vi "Control Panel.vi"(8 "error in (no error)":errorcluster, 11 "Fake Analog Output in":refnum<class "Analog Output.lvclass">) -> (0 "error out":errorcluster, 3 "Fake Analog Output out":refnum<class "Analog Output.lvclass">)   [LabVIEW 2017, in "Analog Output.lvclass"]
doc: "(Dynamic) A user-level application that simulates the physical front panel of the Instrument. Provide the user with buttons to manually control features of the instrument, and provide indicators of its current state."
uses:
  Analog Output.lvclass
  Analog Output.lvclass/Analog Output.ctl
  <vilib>/DAQmx/write.llb/DAQmx Write (Analog DBL 1Chan 1Samp).vi
  <vilib>/DAQmx/miscellaneous.llb/DAQmx Fill In Error Info.vi
  Utility Classes/Scannable/Scannable.lvclass
  <resource>/objmgr/daqmx.rc
panel:
  in  "Copy actual to set":bool
  in  "Populate fields with member data":bool
  out "Ch1 voltage":dbl[unit]
  out "Ch1 lower limit":dbl[unit]
  out "Ch1 upper limit":dbl[unit]
  out "Ch0 voltage":dbl[unit]
  out "Ch0 lower limit":dbl[unit]
  out "Ch0 upper limit":dbl[unit]
  in  "Set Ch1 Voltage":bool
  in  "Set Ch0 Voltage":bool
  in  "Ch1 voltage set":dbl[unit]
  in  "Ch1 lower limit set":dbl[unit]
  in  "Ch1 upper limit set":dbl[unit]
  in  "Ch0 voltage set":dbl[unit]
  in  "Ch0 lower limit set":dbl[unit]
  in  "Ch0 upper limit set":dbl[unit]
  in  "Set Parameters":bool
  in  "Read to Control":bool
  in  "Read Parameters":bool
  in  "stop":bool
  # "We cannot read in the currently set voltage values !"
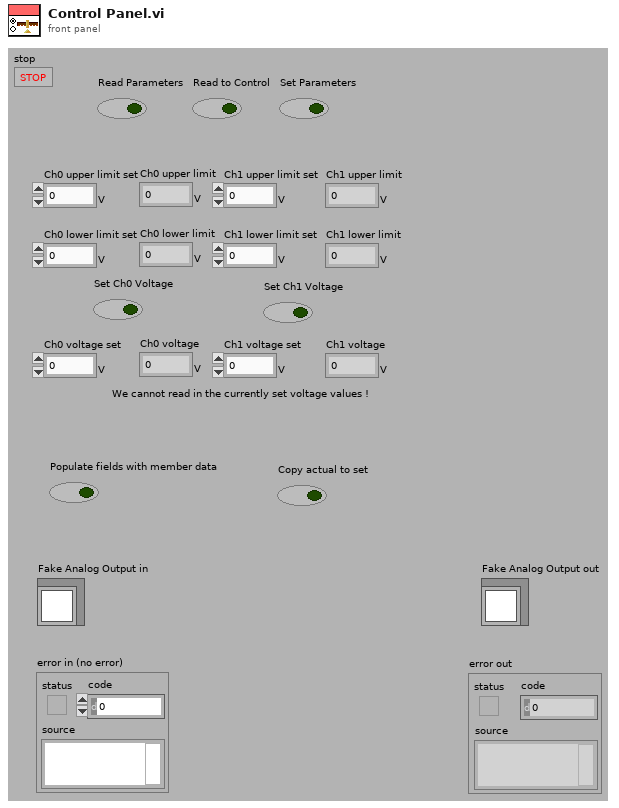
[diagram p1: front panel]
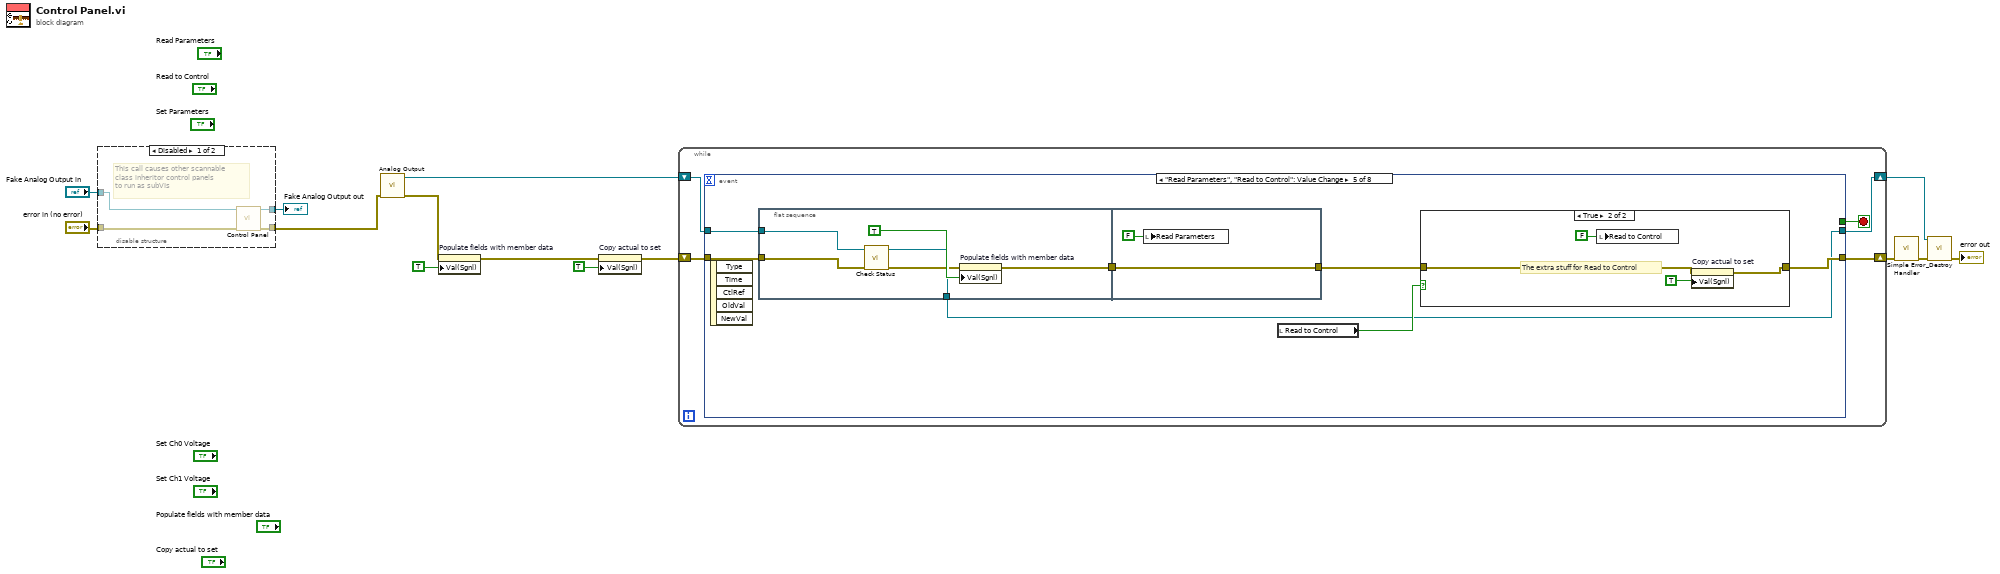
[diagram p0: block diagram]
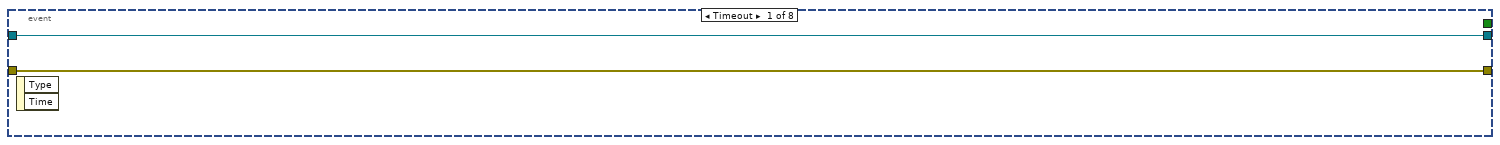
[diagram p3: hidden frame]
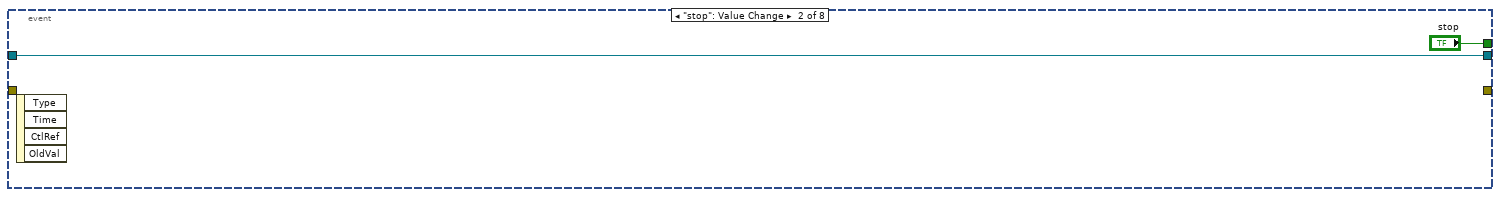
[diagram p4: hidden frame]
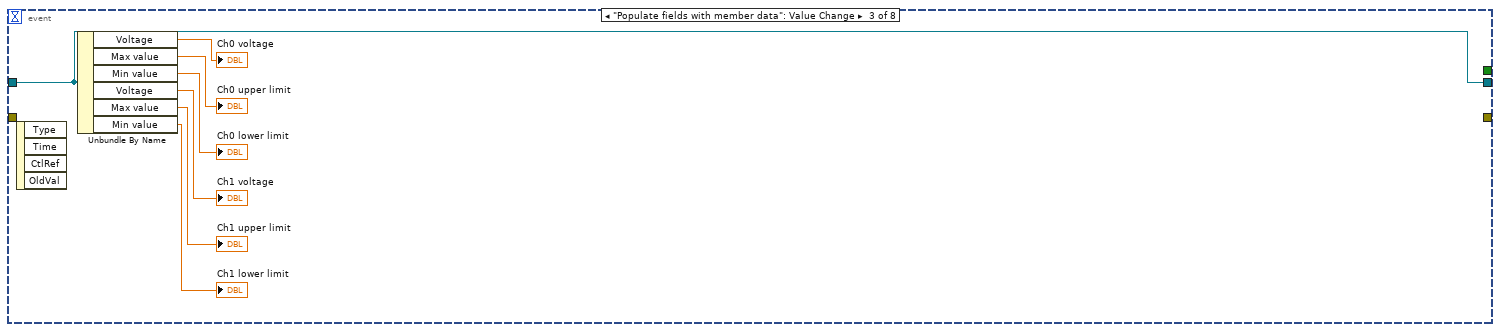
[diagram p5: hidden frame]
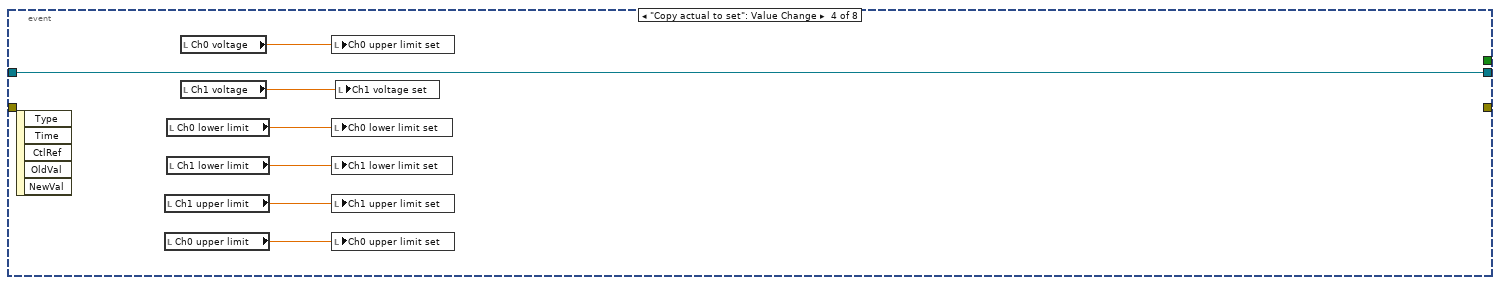
[diagram p6: hidden frame]
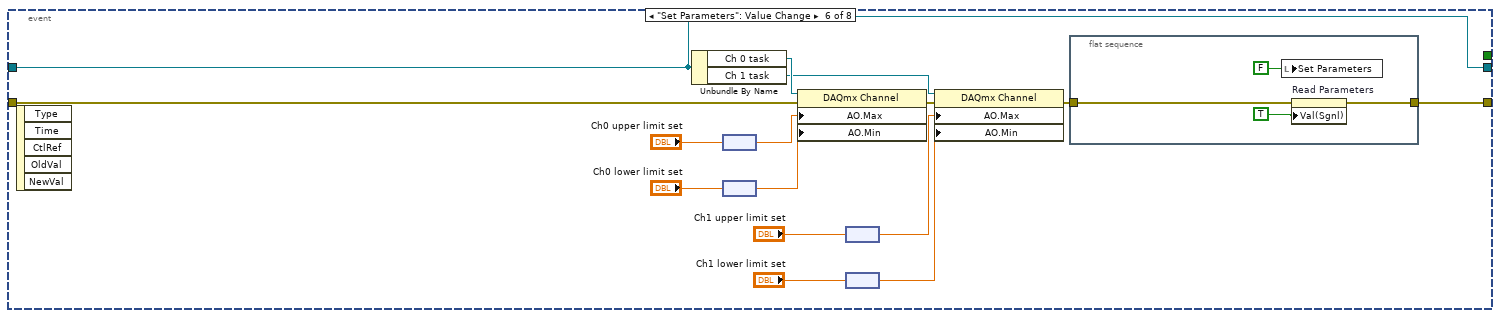
[diagram p8: hidden frame]
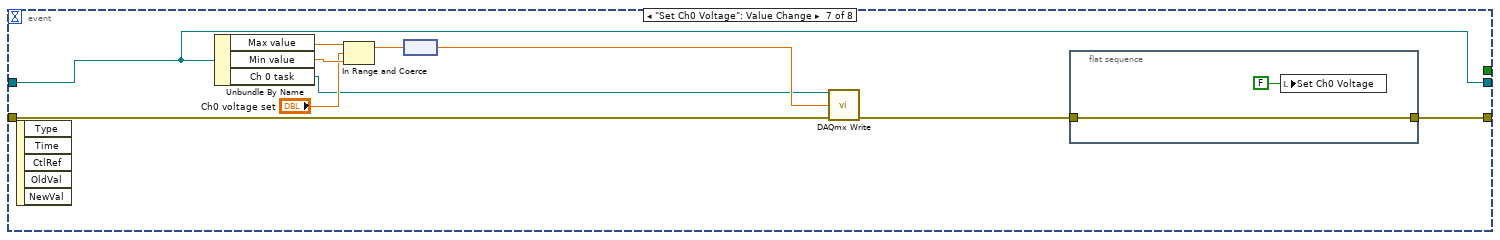
[diagram p9: hidden frame]
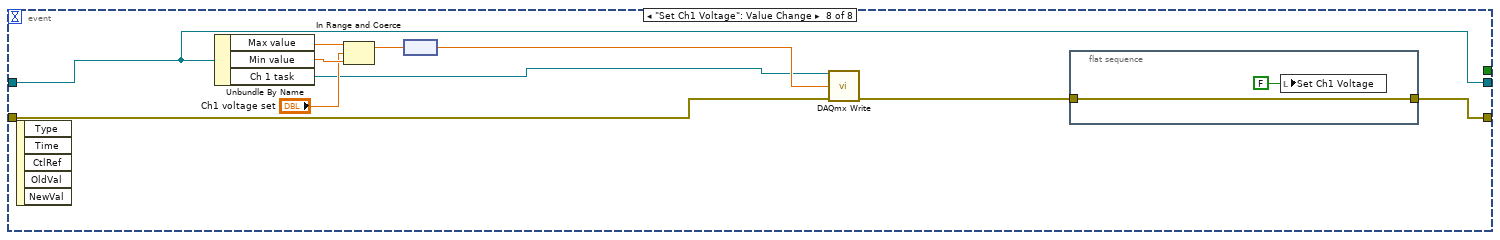
[diagram p10: hidden frame]
diagram:
  n1 = disable-structure shown="Disabled" {
    disable-tunnel: [w18 w20] -> w14
    disable-tunnel: "error in (no error)" -> [w17 w19]
    disable-tunnel: "Fake Analog Output in" -> [w16 w20]
    disable-tunnel: [w15 w19] -> w11
    frame Disabled {
      # "This call causes other scannable\nclass inheritor control panels\nto run as subVIs"
      n2 = call-parent "Control Panel.vi"("error in (no error)"=w17, "Instrument in"=w16) -> ("error out"=w15:errorcluster, "Instrument out"=w18:refnum<class "Analog Output.lvclass">)  [unwired: 8 in]
    }
    frame Enabled {
    }
  }
  "Fake Analog Output out" <- w14
  n3 = call "Analog Output.vi"("error in (no error)"=w11) -> ("error out"=w9:errorcluster, "Analog Output out"=w3:refnum<class "Analog Output.lvclass">)  [unwired: 9 in]
  n4 = property on="Populate fields with member data" class="Bool (strict)"(error in=w9, "Val(Sgnl)"=TRUE ("Value (Signaling)")) -> (error out=w7:errorcluster)  [unwired: 1 in, 1 out]
  n5 = property on="Copy actual to set" class="Bool (strict)"(error in=w7, "Val(Sgnl)"=TRUE ("Value (Signaling)")) -> (error out=w6:errorcluster)  [unwired: 1 in, 1 out]
  n6 = while {
    shift-right: [w23] -> w2
    shift-left: w3 -> [w24]
    shift-right: [w22] -> w1
    shift-left: w6 -> [w25]
    stop <- w21 stop-if-true
    n7 = event shown="[4] \"Read Parameters\", \"Read to Control\": Value Change" {
      selector: _ -> [_ _ _ _ _ _ _ _]
      dyn-events: _ -> [_ _ _ _ _ _ _ _]
      timeout: _ -> [_ _ _ _ _ _ _ _]
      tunnel: [w27 _ _ _ w45 w69 w91 w103] -> w22
      tunnel: w25 -> [w27 _ _ _ w49 w78 w85 w97]
      tunnel: w24 -> [w26 w28 w36 w37 w50 w68 w90 w98]
      tunnel: [w26 w28 w36 w37 w44 w68 w90 w98] -> w23
      tunnel: [_ "stop" _ _ _ _ _ _] -> w21
      event Timeout {
        n8 = event-data() -> ()  [unwired: 1 in, 2 out]
      }
      event "stop": Value Change {
        n9 = event-data() -> ()  [unwired: 1 in, 4 out]
      }
      event "Populate fields with member data": Value Change {
        n10 = event-data() -> ()  [unwired: 1 in, 4 out]
        n11 = Unbundle By Name(w36) -> ("Voltage"=→"Ch0 voltage":dbl[unit], "Max value"=→"Ch0 upper limit":dbl[unit], "Min value"=→"Ch0 lower limit":dbl[unit], "Voltage"=→"Ch1 voltage":dbl[unit], "Max value"=→"Ch1 upper limit":dbl[unit], "Min value"=→"Ch1 lower limit":dbl[unit])
      }
      event "Copy actual to set": Value Change {
        n12 = event-data() -> ()  [unwired: 1 in, 5 out]
        n13 = local read "Ch1 upper limit"() -> (w39:dbl[unit])
        n14 = local read "Ch0 upper limit"() -> (w42:dbl[unit])
        n15 = local read "Ch0 lower limit"() -> (w43:dbl[unit])
        n16 = local read "Ch1 lower limit"() -> (w40:dbl[unit])
        n17 = local read "Ch0 voltage"() -> (w41:dbl[unit])
        n18 = local read "Ch1 voltage"() -> (w38:dbl[unit])
        n19 = local write "Ch0 upper limit set"(w41) -> ()
        n20 = local write "Ch0 lower limit set"(w43) -> ()
        n21 = local write "Ch1 lower limit set"(w40) -> ()
        n22 = local write "Ch1 upper limit set"(w39) -> ()
        n23 = local write "Ch0 upper limit set"(w42) -> ()
        n24 = local write "Ch1 voltage set"(w38) -> ()
      }
      event "Read Parameters", "Read to Control": Value Change {
        n25 = event-data() -> ()  [unwired: 1 in, 5 out]
        n26 = flat-sequence {
          tunnel: w50 -> [w61]
          tunnel: w49 -> [w60]
          tunnel: [w57] -> w48
          tunnel: [w56] -> w44
          tunnel: [w62] -> w46
          tunnel: w48 -> [w62]
          frame #0 {
            n27 = call-dynamic "Check Status.vi"("error in (no error)"=w60, "Analog Output in"=w61) -> ("error out"=w58:errorcluster, "Analog Output out"=w56:refnum<class "Analog Output.lvclass">)  [unwired: 6 in, 2 out]
            n28 = property on="Populate fields with member data" class="Bool (strict)"(error in=w58, "Val(Sgnl)"=TRUE ("Value (Signaling)")) -> (error out=w57:errorcluster)  [unwired: 1 in, 1 out]
          }
          frame #1 {
            n29 = local write "Read Parameters"(FALSE ("Read Parameters")) -> ()
          }
        }
        n30 = local read "Read to Control"() -> (w47:bool)
        n31 = case shown="True" w47 {
          tunnel: w46 -> [w51 w54]
          tunnel: [w51 w53] -> w45
          frame False {
          }
          frame True {
            # "The extra stuff for Read to Control"
            n32 = local write "Read to Control"(FALSE ("Read to Control")) -> ()
            n33 = property on="Copy actual to set" class="Bool (strict)"(error in=w54, "Val(Sgnl)"=TRUE ("Value (Signaling)")) -> (error out=w53:errorcluster)  [unwired: 1 in, 1 out]
          }
        }
      }
      event "Set Parameters": Value Change {
        n34 = event-data() -> ()  [unwired: 1 in, 5 out]
        n35 = Unbundle By Name(w68) -> ("Ch 0 task"=w67:refnum<k21>, "Ch 1 task"=w66:refnum<k21>)
        n36 = node("Ch0 upper limit set") -> (w76:dbl)
        n37 = node("Ch0 lower limit set") -> (w72:dbl)
        n38 = property class="DAQmx Channel"(reference=w67, error in=w78, "AO.Max"=w76, "AO.Min"=w72) -> (error out=w65:errorcluster)  [unwired: 1 out]
        n39 = node("Ch1 upper limit set") -> (w71:dbl)
        n40 = node("Ch1 lower limit set") -> (w70:dbl)
        n41 = property class="DAQmx Channel"(reference=w66, error in=w65, "AO.Max"=w71, "AO.Min"=w70) -> (error out=w64:errorcluster)  [unwired: 1 out]
        n42 = flat-sequence {
          tunnel: w64 -> [w81]
          tunnel: [w80] -> w69
          frame #0 {
            n43 = local write "Set Parameters"(FALSE ("Set Parameters")) -> ()
            n44 = property on="Read Parameters" class="Bool (strict)"(error in=w81, "Val(Sgnl)"=TRUE ("Value (Signaling)")) -> (error out=w80:errorcluster)  [unwired: 1 in, 1 out]
          }
        }
      }
      event "Set Ch0 Voltage": Value Change {
        n45 = event-data() -> ()  [unwired: 1 in, 5 out]
        n46 = Unbundle By Name(w90) -> ("Max value"=w89:dbl[unit], "Min value"=w88:dbl[unit], "Ch 0 task"=w84:refnum<k21>)
        n47 = In Range and Coerce(upper limit=w89, x="Ch0 voltage set", lower limit=w88) -> (coerced(x)=w86:dbl[unit])  [unwired: 1 out]
        n48 = node(w86) -> (w92:dbl)
        n49 = call-poly <vilib>:"DAQmx Write.vi"("task/channels in"=w84, "data"=w92, "error in"=w85) -> ("error out"=w83:errorcluster)  [unwired: 10 in, 2 out]
        n50 = flat-sequence {
          tunnel: [w93] -> w91
          tunnel: w83 -> [w93]
          frame #0 {
            n51 = local write "Set Ch0 Voltage"(FALSE ("Set Ch0 Voltage")) -> ()
          }
        }
      }
      event "Set Ch1 Voltage": Value Change {
        n52 = event-data() -> ()  [unwired: 1 in, 5 out]
        n53 = Unbundle By Name(w98) -> ("Max value"=w102:dbl[unit], "Min value"=w101:dbl[unit], "Ch 1 task"=w96:refnum<k21>)
        n54 = In Range and Coerce(upper limit=w102, x="Ch1 voltage set", lower limit=w101) -> (coerced(x)=w100:dbl[unit])  [unwired: 1 out]
        n55 = node(w100) -> (w104:dbl)
        n56 = call-poly <vilib>:"DAQmx Write.vi"("task/channels in"=w96, "data"=w104, "error in"=w97) -> ("error out"=w95:errorcluster)  [unwired: 10 in, 2 out]
        n57 = flat-sequence {
          tunnel: [w105] -> w103
          tunnel: w95 -> [w105]
          frame #0 {
            n58 = local write "Set Ch1 Voltage"(FALSE ("Set Ch1 Voltage")) -> ()
          }
        }
      }
    }
  }
  n59 = call <vilib>:"Simple Error Handler.vi"("error in (no error)"=w1) -> ("error out"=w5:errorcluster)  [unwired: 1 in, 7 out]
  n60 = call-dynamic "_Destroy.vi"("error in (no error)"=w5, "Analog Output in"=w2) -> ("error out"=→"error out":errorcluster)  [unwired: 9 out]
